vi "Event Ctr, Falling Edge.vi"() -> ()   [LabVIEW 2016]
doc: "This VI contains an event counter that increments on every falling edge of the input trigger signal. To reset the value of the counter, push the reset button.\n\nThe trigger address is set to PB1 and reset address to PB2 on the evaluation board. The 8-bit count will be shown on the front panel indicator below as well as on the evaluation board's eight LEDs (represented in binary)."
uses:
  <vilib>/Platform/TimedLoop/XDataNode/timing_clust.ctl
  <vilib>/Platform/TimedLoop/XDataNode/nitl_modes.ctl
  <vilib>/Platform/TimedLoop/XDataNode/wakeup.ctl
  <vilib>/rvi/Emulation/niFpgaSctlEmulationGetInTimedLoop.vi
  <vilib>/rvi/Emulation/niFpgaEmulationReportErrorSimple.vi
  <vilib>/rvi/Emulation/niFpgaGetClockAttributes.vi
  <vilib>/rvi/Emulation/niFpgaCriticalErrorInLSC.vi
  <vilib>/rvi/eio/common/nirviEmuTemplateMethod_errors.vi
  <vilib>/Platform/TimedLoop/XDataNode/XDataNode.xnode
  <vilib>/eio/EIONode/EIONode.xnode
  <vilib>/Platform/TimedLoop/XDataNode/XDNodeRunTimeDep.lvlib
panel:
  in  "stop":bool
  out "8-bit Count":u8
  # "This VI contains an event counter that increments on every falling edge of the input trigger signal.  To reset the value of the counter, push the reset button. The trigger address is set to PB1 and reset address to PB2 on the evaluation board. The 8-bit count will be shown on the front panel indicator below as well as on the evaluation board's six LEDs, where only the first six binary digits of the 8-bit count are displayed."
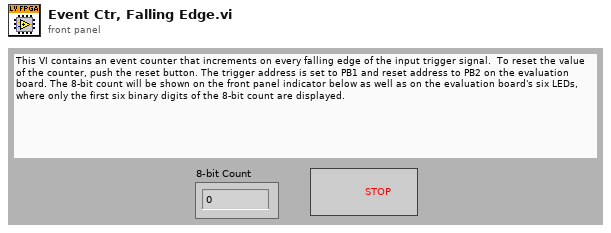
[diagram p1: front panel]
types:
  T1 = typedef "XDNodeRunTimeDep.lvlib/timing_clust.ctl" = cluster{"Expected End [f-1]":u64, "Actual End [f-1]":u64, "Finished Late? [f-1]":bool, "Expected End [i-1]":u64, "Actual End [i-1]":u64, "Finished Late? [i-1]":bool, "Expected Start [i]":u64, "Actual Start [i]":u64, "Expected Start [f]":u64, "Actual Start [f]":u64, "Source Name":string, "Structure Name":string, "Period":i64, "Deadline":i64, "Offset":i64, "Start":i64, "Priority":i32, "Timeout":i32, "Mode":T2, "Wakeup Reason":T3, "Error":errorcluster, "Source Type":string, "Secondary Source Type":string, "Global End Time":u64, "Global Start Time":u64, "Frame Duration":u64, "Iteration Duration":u64, "Assigned CPU":i32, "I/O Scan Engine Mode":u32}
  T2 = typedef "XDNodeRunTimeDep.lvlib/nitl_modes.ctl" = enum32{"No Change", "Process missed periods, maintain original phase", "Discard missed periods, maintain original phase", "Process missed periods, ignore original phase", "Discard missed periods, ignore original phase"}
  T3 = typedef "XDNodeRunTimeDep.lvlib/wakeup.ctl" = enum32{"Normal", "Aborted", "Asynchronous wakeup", "Timing source error", "Timed loop error", "Timeout"}
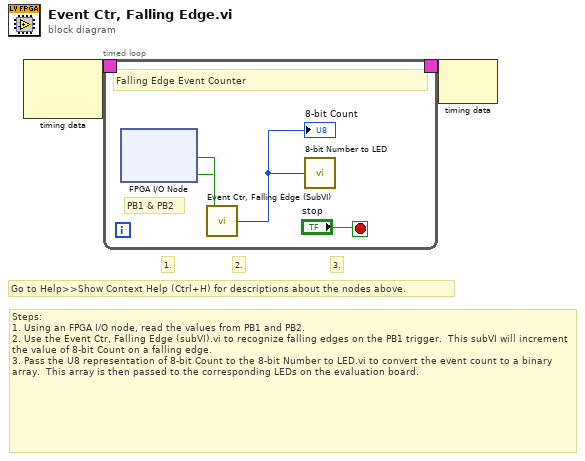
[diagram p0: block diagram]
diagram:
  # "Go to Help>>Show Context Help (Ctrl+H) for descriptions about the nodes above."
  # "1."
  # "3."
  # "2."
  # "Steps:\n1. Using an FPGA I/O node, read the values from PB1 and PB2.\n2. Use the Event Ctr, Falling Edge (subVI).vi to recognize falling edges on the PB1 trigger.  This subVI will increment the value of 8-bit Count on a falling edge.\n3. Pass the U8 representation of 8-bit Count to the 8-bit Number to LED.vi to convert the event count to a binary array.  This array is then passed to the corresponding LEDs on the evaluation board."
  n1 = node-c288() -> (w1:T1)  [unwired: 2 out]
  n2 = timed-loop {
    timing-out: [_] -> w2
    timing: w1 -> [_]
    stop <- "stop" stop-if-true
    # "PB1 & PB2"
    # "Falling Edge Event Counter"
    n3 = xnode "FPGA I/O Node"() -> ("DIO12"=w4:bool, "DIO13"=w3:bool)  [unwired: 2 in, 2 out]
    n4 = call "Event Ctr, Falling Edge (SubVI).vi"("Reset"=w3, "Trigger"=w4) -> ("8-bit Count (0-63)"=w5:u8)
    "8-bit Count" <- w5
    n5 = call "8-bit Number to LED.vi"("6-bit Unsigned\n Number (0-63)"=w5) -> ()  [unwired: 1 out]
  }
  n6 = node-c288(w2) -> ()  [unwired: 1 out]
